vi "Version Check.vi"(8 "에러 입력":errorcluster caption="에러 입력(에러 없음)") -> (0 "에러 출력":errorcluster, 1 "MCT 업데이트?":bool, 2 "FTP 업데이트?":bool, 4 "MCT 로컬버전":string, 5 "Updater 로컬버전":string, 6 "MCT 서버버전":string, 7 "Updater 서버버전":string)   [LabVIEW 2020]
uses:
  Controls/Cmd_Read Query.ctl
  Polymorph/ini Ctrl_Str.vi
  <vilib>/addons/database/NI_Database_API.lvlib
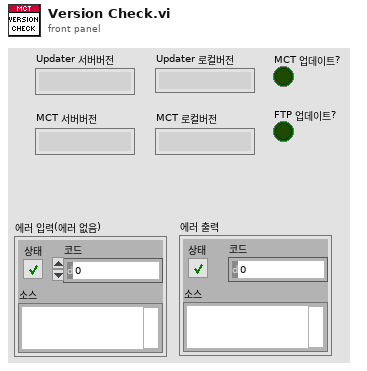
[diagram p1: front panel]
types:
  T1 = typedef "Cmd_Read Query.ctl" = enum16{"교정자 이름 얻기", "인증교정자 얻기", "기술책임자 얻기", "기책부책 얻기", "등록번호 얻기", "등록정보 얻기", "업체정보 얻기", "교정일자(CAMAS) 얻기", "교정일자(CALSTD) 얻기", "교정환경 얻기", "교정절차서 목록 얻기", "교정절차서명 얻기", "교정절차 목록얻기", "교정절차 얻기", "PROC 교정절차 얻기", "PROC SPEC 얻기", "교정절차(Func별) 얻기", "교정절차(Func_ext별) 얻기", "기관코드 얻기", "교정기능(세부분류) 얻기", "교정기능(모델) 얻기", "교정기능 목록 얻기", "교정기능 명칭 얻기", "교정기능 항목명칭 얻기", "DB (사용기준기) 얻기", "DB (기준기이름) 얻기", "DB (기준기이름목록) 얻기", "DB (기준기목록) 얻기", "DB (기준기값) 얻기", "DB (CMC) 얻기", "DB (FUNC) 얻기", "DB (CALNAME) 얻기", "DB (STDNAME) 얻기", "DB (SPEC) 얻기", "모델(항목전체) 얻기", "모델(최대범위) 얻기", "모델(최소범위) 얻기", "모델(최대최소) 얻기", "모델(범위조건) 얻기", "모델(등록요청) 얻기", "모델(형식별) 얻기", "모델(조건별) 얻기", "모델(모델검색) 얻기", "세부분류 목록 얻기", "기준기등록리스트 얻기", "STD Cal Date Check", "DB등록일자 얻기", "적용항목 얻기", "기타정보 얻기", "기준기요청 얻기", "서버버전 얻기"}
  T2 = typedef "NI_Database_API.lvlib/Conn ObjectReference.ctl" = refnum<k1>
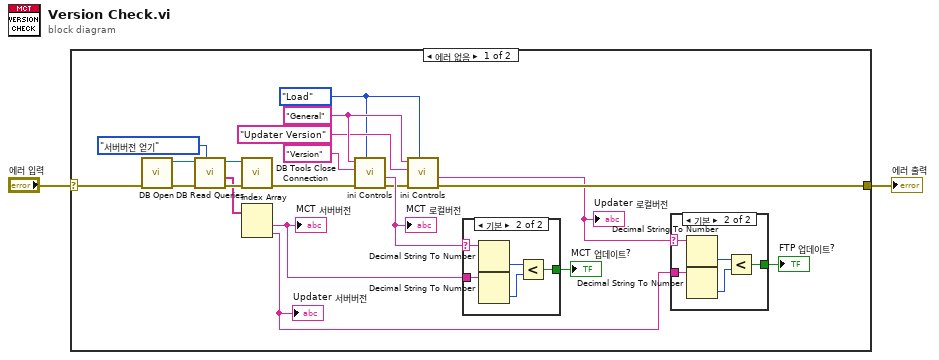
[diagram p0: block diagram]
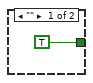
[diagram p2: hidden frame]
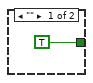
[diagram p3: hidden frame]
diagram:
  n1 = case shown="에러 없음" "에러 입력" {
    selector: "에러 입력" -> [w20 w35]
    tunnel: [w8 w35] -> w2
    frame No Error {
      w10 = enum16{"Save", "Load"}."Load" ("Select")
      w12 = "General" ("section")
      n2 = call "DB Open.vi"("에러 입력"=w20) -> ("에러 출력"=w18:errorcluster, "참조 번호 출력"=w19:T2)  [unwired: 9 in]
      n3 = call "DB Read Queries.vi"("Query Command"=Cmd_Read_Query."서버버전 얻기", "에러 입력(에러 없음)"=w18, "참조 번호 입력"=w19) -> ("에러 출력"=w16:errorcluster, "Data (0번행)"=w14:string[], "참조 번호 출력"=w17:T2)  [unwired: 4 in, 2 out]
      n4 = call <vilib>:"DB Tools Close Connection.vi"("error in (no error)"=w16, "connection reference"=w17) -> ("error out"=w7:errorcluster)  [unwired: 5 in]
      n5 = Index Array(array=w14) -> (element #1=w13:string, element #2=w3:string)  [unwired: 2 in]
      "MCT 서버버전" <- w13
      "Updater 서버버전" <- w3
      n6 = call-poly "ini Controls.vi"("Select"=w10, "에러 입력"=w7, "키"="Version" ("key"), "섹션"=w12) -> ("에러 출력"=w9:errorcluster, "값"=w21:string)  [unwired: 5 in, 1 out]
      "MCT 로컬버전" <- w21
      n7 = call-poly "ini Controls.vi"("Select"=w10, "에러 입력"=w9, "키"="Updater Version" ("key"), "섹션"=w12) -> ("에러 출력"=w8:errorcluster, "값"=w4:string)  [unwired: 5 in, 1 out]
      "Updater 로컬버전" <- w4
      n8 = case shown="기본" w21 {
        selector: w21 -> [_ w30]
        tunnel: w13 -> [_ w34]
        tunnel: [TRUE w31] -> w6
        frame "" {
        }
        frame Default {
          n9 = Decimal String To Number(string=w30) -> (number=w32:i32)  [unwired: 2 in, 1 out]
          n10 = Decimal String To Number(string=w34) -> (number=w33:i32)  [unwired: 2 in, 1 out]
          n11 = Less?(x=w32, y=w33) -> (x < y?=w31:bool)
        }
      }
      "MCT 업데이트?" <- w6
      n12 = case shown="기본" w4 {
        selector: w4 -> [_ w24]
        tunnel: w3 -> [_ w28]
        tunnel: [TRUE w25] -> w5
        frame "" {
        }
        frame Default {
          n13 = Decimal String To Number(string=w24) -> (number=w26:i32)  [unwired: 2 in, 1 out]
          n14 = Decimal String To Number(string=w28) -> (number=w27:i32)  [unwired: 2 in, 1 out]
          n15 = Less?(x=w26, y=w27) -> (x < y?=w25:bool)
        }
      }
      "FTP 업데이트?" <- w5
    }
    frame Error {
    }
  }
  "에러 출력" <- w2
